vi "Decimal String to Binary number.vi"(8 "error in (no error)":errorcluster, 11 "Excel Data":string[][](array[string])) -> (0 "error out":errorcluster, 3 "Excel Binary Data":i16[][](array[numeric]))   [LabVIEW 2016, in "User Interface.lvlib"]
uses:
  User Interface.lvlib
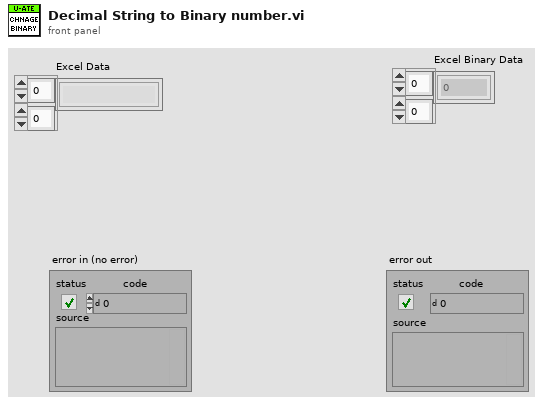
[diagram p1: front panel]
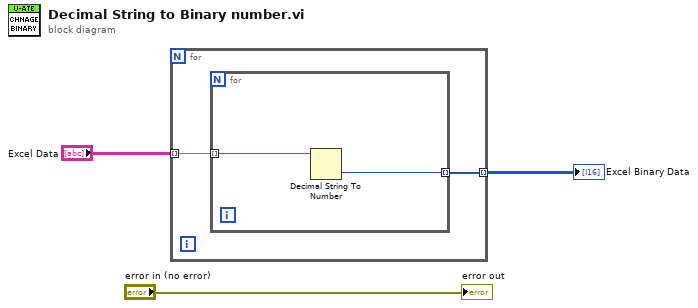
[diagram p0: block diagram]
diagram:
  n1 = for {
    tunnel: "Excel Data" -> [w5] mode=indexing
    tunnel: [w4] -> w1 mode=indexing
    n2 = for {
      tunnel: w5 -> [w7] mode=indexing
      tunnel: [w6] -> w4 mode=indexing
      n3 = Decimal String To Number(string=w7) -> (number=w6:i32)  [unwired: 2 in, 1 out]
    }
  }
  "Excel Binary Data" <- w1
  "error out" <- "error in (no error)"
